vi "AlliGator Build Phasor Calibration Map.vi"(7 "Decay Metadata Array":T1[](array[typedef]) {"# Folds" min=1; "ROI Descriptor"."Contours"."Type" items=["No Selection", "Point", "Line", "Rectangle", "Oval", "Polygon", "Freehand Region", "Annulus", "Unused2", "Unused3", "Broken Line", "Freehand Line", "Rotated Rectangle"]}, 8 "Error In":errorcluster, 9 "Calibration Lifetime":dbl[unit]=1e-09, 10 "Phasor Frequency":dbl[unit]=80000000.0, 11 "Uncalibrated Phasors":T9[](array[typedef])) -> (0 "Error Out":errorcluster, 1 "Valid Map?":bool, 2 "Duplicate ROIs?":bool, 3 "Phasor Calibration Map":T8={"Phasor Frequency"=80000000.0, "Calibration Lifetime"=1e-09, "ROI Centers"=[], "ROI Descriptors"=[], "Map Resolution X"=0, "Map Resolution Y"=0, "z Array"=[]} {"ROI Descriptors"."Contours"."Type" items=["No Selection", "Point", "Line", "Rectangle", "Oval", "Polygon", "Freehand Region", "Annulus", "Unused2", "Unused3", "Broken Line", "Freehand Line", "Rotated Rectangle"]})   [LabVIEW 2021, in "AlliGator Phasor Calibration.lvlib"]
doc: "Packages the provided <B>Uncalibrated Phasors</b> as a <B>Phasor Calibration Map</B>."
uses:
  AlliGator Phasor Calibration.lvlib
  Phasor/Phasor (g, s).ctl
  Phasor/Phasor Calibration Map v2.ctl
  Phasor Graph/AlliGator Decay Metadata v3.ctl
  Decay Analysis/Decay Preprocessing/AlliGator Decay Background Subtraction Info.ctl
  Decay Analysis/Decay Preprocessing/AlliGator Baseline Subtraction Method.ctl
  Graphs/XY Graph/XY Graph Plot Shift Parameters.ctl
  Graphs/XY Graph/XY Graph Plot Shift Method.ctl
  Decay Analysis/Decay Preprocessing/AlliGator Decay Extrapolation Parameters.ctl
  c1f5ce2d-1d26-483e-b821-1bd9bf197e8c.vi
  Phasor/Phasor.lvlib
  Utilities/Utilities.lvlib
  Phasor Graph/AlliGator Phasor Graph.lvlib
  Decay Analysis/Decay Preprocessing/AlliGator Decay Preprocessing.lvlib
  Graphs/XY Graph/XY Graph Add-Ons.lvlib
panel:
  # "see the AlliGator License on the block diagram (Ctrl+E or Window:Show Block Diagram)"
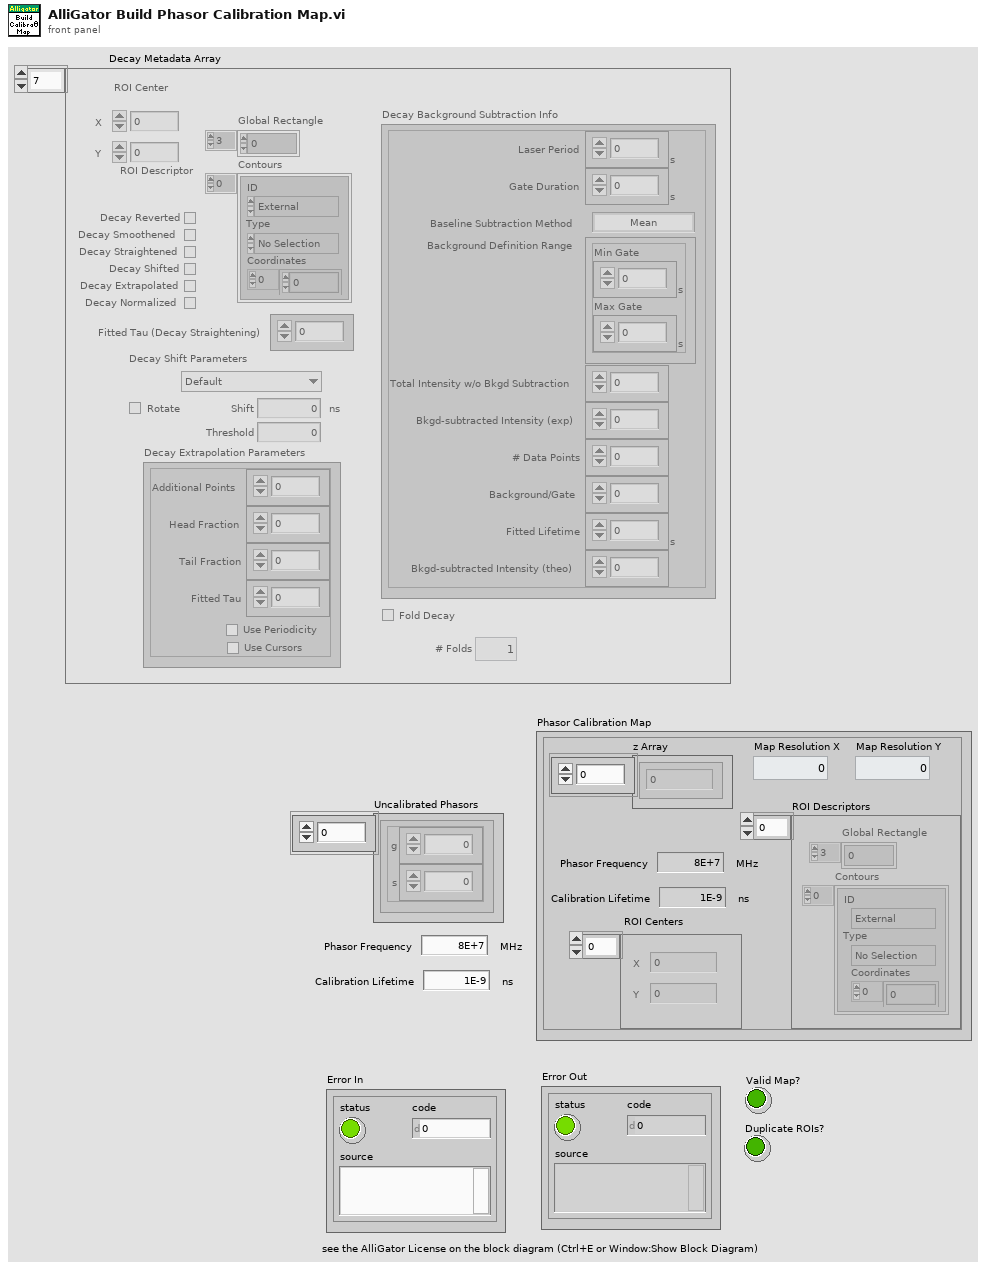
[diagram p1: front panel]
types:
  T1 = typedef "AlliGator Phasor Graph.lvlib/AlliGator Decay Metadata v3.ctl" = cluster{"ROI Descriptor":T2, "ROI Center":cluster{"X":i32, "Y":i32}, "Decay Background Subtraction Info":T3, "Decay Reverted":bool, "Decay Smoothened":bool, "Decay Straightened":bool, "Fitted Tau (Decay Straightening)":dbl, "Decay Shift Parameters":T5, "Decay Shifted":bool, "Decay Extrapolated":bool, "Decay Extrapolation Parameters":T7, "Decay Normalized":bool, "Fold Decay":bool, "# Folds":u32}
  T2 = typedef "ROI Descriptor" = cluster{"Global Rectangle":i32[], "Contours":cluster{"ID":enum32{"External", "Internal"}, "Type":u32, "Coordinates":i32[]}[]}
  T3 = typedef "AlliGator Decay Preprocessing.lvlib/AlliGator Decay Background Subtraction Info.ctl" = cluster{"Laser Period":dbl[unit], "Gate Duration":dbl[unit], "Baseline Subtraction Method":T4, "Background Definition Range":cluster{"Min Gate":dbl[unit], "Max Gate":dbl[unit]}, "Total Intensity w/o Bkgd Subtraction":dbl, "Bkgd-subtracted Intensity (exp)":dbl, "# Data Points":i32, "Background/Gate":dbl, "Fitted Lifetime":dbl[unit], "Bkgd-subtracted Intensity (theo)":dbl}
  T4 = typedef "AlliGator Decay Preprocessing.lvlib/AlliGator Baseline Subtraction Method.ctl" = enum16{"Mean", "Min", "Square Gated Single-Exponential", "File", "Constant"}
  T5 = typedef "XY Graph Add-Ons.lvlib/XY Graph Plot Shift Parameters.ctl" = cluster{"Type":T6, "Shift":dbl[unit], "Threshold":dbl, "Rotate":bool}
  T6 = typedef "XY Graph Add-Ons.lvlib/XY Graph Plot Shift Method.ctl" = enum16{"Default", "CFD", "Threshold", "Cross-Correlation"}
  T7 = typedef "AlliGator Decay Preprocessing.lvlib/AlliGator Decay Extrapolation Parameters.ctl" = cluster{"Additional Points":u32, "Head Fraction":dbl, "Fitted Tau":dbl, "Use Periodicity":bool, "Use Cursors":bool, "Tail Fraction":dbl}
  T8 = typedef "Phasor.lvlib/Phasor Calibration Map v2.ctl" = cluster{"Phasor Frequency":dbl[unit], "Calibration Lifetime":dbl[unit], "ROI Centers":cluster{"X":i32, "Y":i32}[], "ROI Descriptors":T2[], "Map Resolution X":i32, "Map Resolution Y":i32, "z Array":cdb[]}
  T9 = typedef "Phasor.lvlib/Phasor (g, s).ctl" = cluster{"g":dbl, "s":dbl}
  T10 = typedef "Phasor.lvlib/Phasor (m, phi).ctl" = cluster{"m":dbl, "phi":dbl}
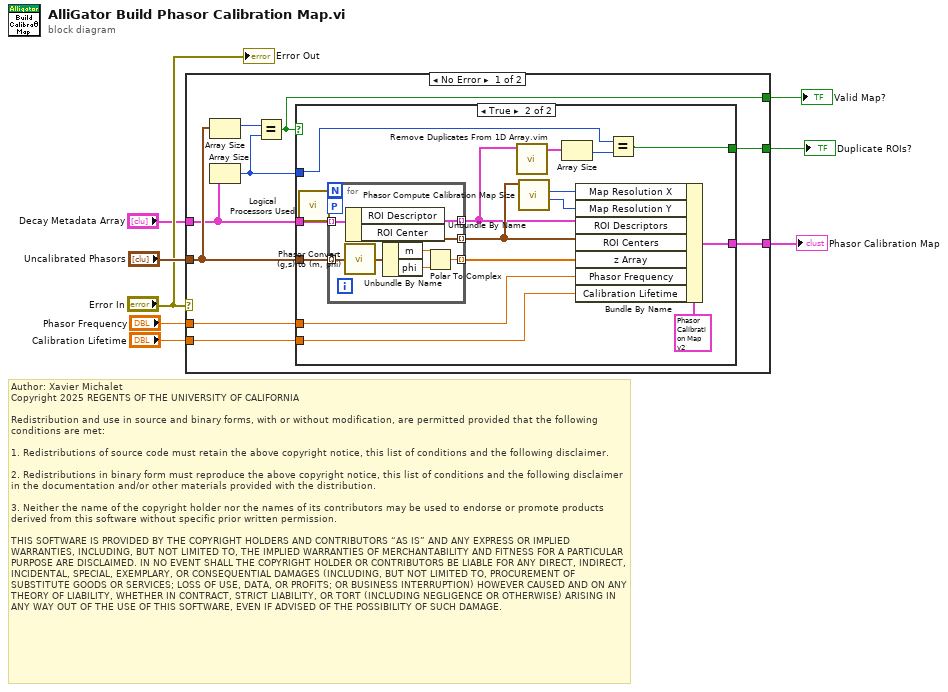
[diagram p0: block diagram]
diagram:
  # "Author: Xavier Michalet\nCopyright 2025 REGENTS OF THE UNIVERSITY OF CALIFORNIA\n\nRedistribution and use in source and binary forms, with or without modification, are permitted provided that the following conditions are met:\n\n1. Redistributions of source code must retain the above copyright notice, this list of conditions and the following disclaimer.\n\n2. Redistributions in binary form must reproduce the above copyright notice, this list of conditions and the following disclaimer in the documentation and/or other materials provided with the distribution.\n\n3. Neither the name of the copyright holder nor the names of its contributors may be used to endorse or promote products derived from this software without specific prior written permission.\n\nTHIS SOFTWARE IS PROVIDED BY THE COPYRIGHT HOLDERS AND CONTRIBUTORS “AS IS” AND ANY EXPRESS OR IMPLIED WARRANTIES, INCLUDING, BUT NOT LIMITED TO, THE IMPLIED WARRANTIES OF MERCHANTABILITY AND FITNESS FOR A PARTICULAR PURPOSE ARE DISCLAIMED. IN NO EVENT SHALL THE COPYRIGHT HOLDER OR CONTRIBUTORS BE LIABLE FOR ANY DIRECT, INDIRECT, INCIDENTAL, SPECIAL, EXEMPLARY, OR CONSEQUENTIAL DAMAGES (INCLUDING, BUT NOT LIMITED TO, PROCUREMENT OF SUBSTITUTE GOODS OR SERVICES; LOSS OF USE, DATA, OR PROFITS; OR BUSINESS INTERRUPTION) HOWEVER CAUSED AND ON ANY THEORY OF LIABILITY, WHETHER IN CONTRACT, STRICT LIABILITY, OR TORT (INCLUDING NEGLIGENCE OR OTHERWISE) ARISING IN ANY WAY OUT OF THE USE OF THIS SOFTWARE, EVEN IF ADVISED OF THE POSSIBILITY OF SUCH DAMAGE."
  n1 = case shown="No Error" "Error In" {
    tunnel: "Phasor Frequency" -> [w17 _]
    tunnel: "Calibration Lifetime" -> [w16 _]
    tunnel: [w15 _] -> w6
    tunnel: "Uncalibrated Phasors" -> [w14 _]
    tunnel: "Decay Metadata Array" -> [w11 _]
    tunnel: [w9 _] -> w2
    tunnel: [w13 _] -> w1
    frame No Error {
      n2 = Array Size(array=w14) -> (size(s)=w12:i32)
      n3 = Array Size(array=w11) -> (size(s)=w10:i32)
      n4 = Equal?(x=w12, y=w10) -> (x = y?=w9:bool)
      n5 = case shown="True" w9 {
        tunnel: w17 -> [_ w33]
        tunnel: w16 -> [_ w32]
        tunnel: [_ w31] -> w15
        tunnel: w14 -> [_ w28]
        tunnel: [_ w18] -> w13
        tunnel: w11 -> [_ w29]
        tunnel: w10 -> [_ w19]
        frame False {
        }
        frame True {
          n6 = call "Logical Processors Used.vi"() -> ("# Logical Processor Used"=w24:i32)  [unwired: 6 in]
          n7 = for {
            tunnel: w28 -> [w41] mode=indexing
            tunnel: w29 -> [w39] mode=indexing
            tunnel: [w38] -> w22 mode=indexing
            tunnel: [w37] -> w27 mode=indexing
            workers-P: w24 -> [_]
            tunnel: [w34] -> w23 mode=indexing
            n8 = call "Phasor Convert (g,s) to (m, phi).vi"("Phasor (g, s)"=w41) -> ("Phasor (m, phi)"=w40:T10)  [unwired: 8 in]
            n9 = Unbundle By Name(w39) -> ("ROI Descriptor"=w38:T2, "ROI Center"=w37:cluster{"X":i32, "Y":i32})
            n10 = Unbundle By Name(w40) -> ("m"=w36:dbl, "phi"=w35:dbl)
            n11 = Polar To Complex(1:w35, 2:w36) -> (0:w34:cdb)
          }
          n12 = call "Remove Duplicates From 1D Array.vim"("array"=w22) -> ("array with duplicates removed"=w21:T2[])  [unwired: 10 in]
          n13 = call "Phasor Compute Calibration Map Size.vi"("Center Coordinates"=w27) -> ("Map Resolution Y"=w25:i32, "Map Resolution X"=w26:i32)  [unwired: 9 in]
          n14 = Array Size(array=w21) -> (size(s)=w20:i32)
          n15 = Bundle By Name(cluster=T8 {"Phasor Frequency"=80000000.0, "Calibration Lifetime"=1e-09, "ROI Centers"=[], "ROI Descriptors"=[], "Map Resolution X"=0, "Map Resolution Y"=0, "z Array"=[]} ("Phasor Reference Plot"), "Map Resolution X"=w26, "Map Resolution Y"=w25, "ROI Descriptors"=w22, "ROI Centers"=w27, "z Array"=w23, "Phasor Frequency"=w33, "Calibration Lifetime"=w32) -> (w31:T8)
          n16 = Equal?(x=w19, y=w20) -> (x = y?=w18:bool)
        }
      }
    }
    frame Error {
    }
  }
  "Phasor Calibration Map" <- w6
  "Valid Map?" <- w2
  "Duplicate ROIs?" <- w1
  "Error Out" <- "Error In"
